vi "DUTBarCode_Parser.vi"(0 "DUT INFO":string, 7 "Rev_suffix":string) -> (1 "Desc":string, 2 "BC_ESN":string="0x00003609B620", 3 "Bar Code":string="TA22240078,0x00003609B620,2224,C.01, Wideband Antenna Module,5083561, RaGE Systems, www.ragesystems.com", 4 "Company":string="RaGE Systems", 6 "BC_MSN":string="TA22240078", 8 "Rage PN":string="5083561", 10 "LotID":string="2224", 13 "BarCodeInfo":string="#RaGE Systems\r\n#Prod_Name: Wideband Antenna Module\r\n#Rage_PN: 5083561\r\n#Revision: C.01\r\n#LotID: 2224\r\n#MSN: TA22240078\r\n#ESN: 0x00003609B620\r\n", 14 "Revision":string="C.01", 15 "rev_c?(t)":bool)   [LabVIEW 2018]
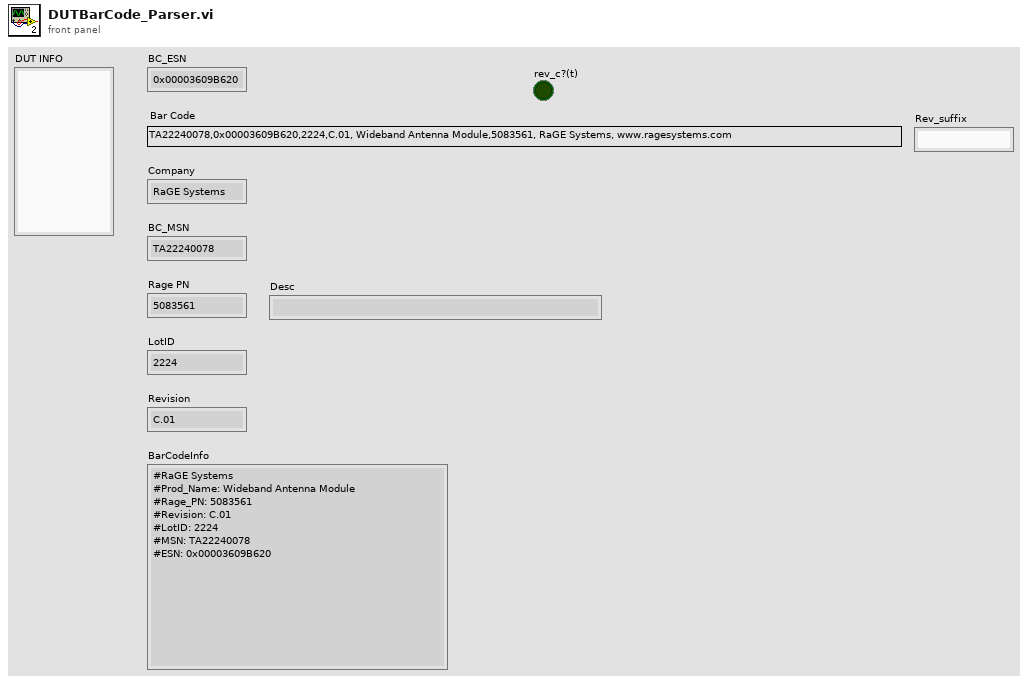
[diagram p1: front panel]
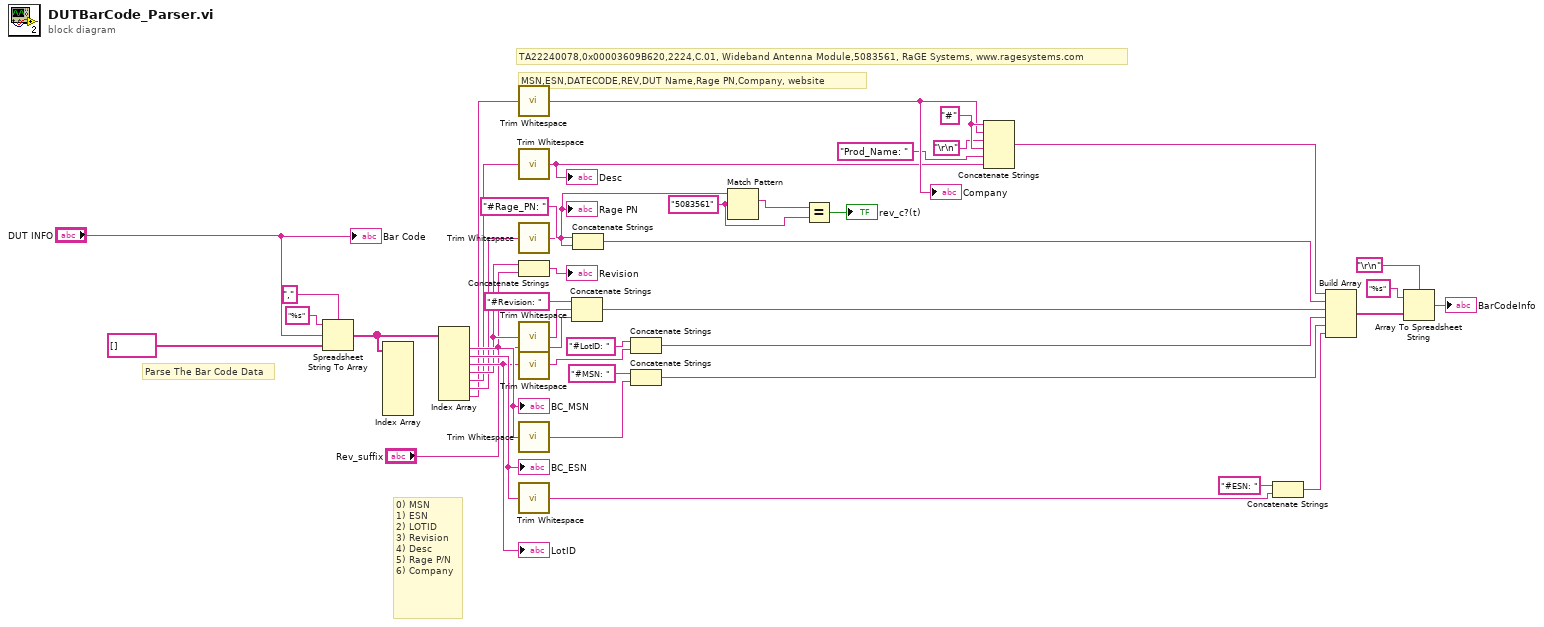
[diagram p0: block diagram]
diagram:
  w2 = "5083561" ("regular expression")
  w37 = "#" ("string")
  # "0) MSN\n1) ESN\n2) LOTID\n3) Revision \n4) Desc\n5) Rage P/N\n6) Company"
  # "MSN,ESN,DATECODE,REV,DUT Name,Rage PN,Company, website"
  # "TA22240078,0x00003609B620,2224,C.01, Wideband Antenna Module,5083561, RaGE Systems, www.ragesystems.com"
  # "Parse The Bar Code Data"
  n1 = Spreadsheet String To Array(delimiter (Tab)=",", format string="%s", spreadsheet string="DUT INFO", array type (2D Dbl)=string[] []) -> (array=w16:string[])
  n2 = Index Array(array=w16) -> ()  [unwired: 7 in, 7 out]
  n3 = Index Array(array=w16) -> (element #1=w15:string, element #2=w14:string, element #3=w13:string, element #4=w12:string, element #5=w10:string, element #6=w11:string, element #7=w9:string)  [unwired: 7 in]
  "BC_MSN" <- w15
  "LotID" <- w13
  "BC_ESN" <- w14
  n4 = call <vilib>:"Trim Whitespace.vi"("string"=w9) -> ("trimmed string"=w35:string)  [unwired: 1 in]
  "Company" <- w35
  n5 = call <vilib>:"Trim Whitespace.vi"("string"=w10) -> ("trimmed string"=w7:string)  [unwired: 1 in]
  "Desc" <- w7
  n6 = call <vilib>:"Trim Whitespace.vi"("string"=w11) -> ("trimmed string"=w4:string)  [unwired: 1 in]
  "Rage PN" <- w4
  n7 = Concatenate Strings(w12, "Rev_suffix") -> (→"Revision":string)
  n8 = call <vilib>:"Trim Whitespace.vi"("string"=w12) -> ("trimmed string"=w38:string)  [unwired: 1 in]
  n9 = call <vilib>:"Trim Whitespace.vi"("string"=w13) -> ("trimmed string"=w39:string)  [unwired: 1 in]
  n10 = call <vilib>:"Trim Whitespace.vi"("string"=w15) -> ("trimmed string"=w40:string)  [unwired: 1 in]
  n11 = call <vilib>:"Trim Whitespace.vi"("string"=w14) -> ("trimmed string"=w41:string)  [unwired: 1 in]
  n12 = Concatenate Strings("#Revision: ", w38, "Rev_suffix") -> (w27:string)
  n13 = Concatenate Strings("#Rage_PN: ", w4) -> (w26:string)
  n14 = Concatenate Strings("#LotID: ", w39) -> (w30:string)
  n15 = Concatenate Strings("#MSN: ", w40) -> (w28:string)
  n16 = Match Pattern(string=w4, regular expression=w2) -> (match substring=w3:string)  [unwired: 1 in, 3 out]
  n17 = Equal?(x=w3, y=w2) -> (x = y?=→"rev_c?(t)":bool)
  n18 = Concatenate Strings(w37, w35, "\r\n", w37, "Prod_Name: " ("string"), w7) -> (w24:string)
  n19 = Concatenate Strings("#ESN: ", w41) -> (w29:string)
  n20 = Build Array(w24, w26, w27, w30, w28, w29) -> (w32:string[])
  n21 = Array To Spreadsheet String(delimiter (Tab)="\r\n", array=w32, 3:"%s" ("format string")) -> (spreadsheet string=→"BarCodeInfo":string)
  "Bar Code" <- "DUT INFO"
